vi "API Tree.vi"   [LabVIEW 2017]
uses:
  user.lib/_NEVSTOP/Communicable State Machine(CSM)/Communicable State Machine.lvlib
  examples/NEVSTOP/Communicable State Machine(CSM)/1. Create a reuse Module/1. Create a reuse Module.lvlib
  examples/NEVSTOP/Communicable State Machine(CSM)/4. Advance Examples/1. Action Workers Example/Action Worker Mode Example.lvlib
  examples/NEVSTOP/Communicable State Machine(CSM)/4. Advance Examples/3. Build-in Error Handling Framework/Build-in Error Handling Framework.lvlib
  examples/NEVSTOP/Communicable State Machine(CSM)/4. Advance Examples/2. Chain of Responsiblility Example/Chain of Responsibility Example.lvlib
  examples/NEVSTOP/Communicable State Machine(CSM)/4. Advance Examples/5. Multi-Loop Module Example/Multi-Loop Module Example.lvlib
  examples/NEVSTOP/Communicable State Machine(CSM)/4. Advance Examples/4. Global Log Filter Example/CSM Global Log Filter Example.lvlib
  user.lib/_NEVSTOP/Communicable State Machine(CSM)/_csmHelper/CSM-Helper.lvclass
  user.lib/_NEVSTOP/Communicable State Machine(CSM)/_csmHelper/lvcsmFile/lvcsm File Support.lvlib
  ddc9829f-1ac7-4767-a110-42ef600eb457.vi
  d8c6dec9-3888-43a3-80fe-73705555c2a7.vi
  user.lib/_NEVSTOP/Communicable State Machine(CSM)/_csmHelper/API with lvcsm Support/CSM-Helper API with lvcsm Support.lvlib
  user.lib/_NEVSTOP/Communicable State Machine(CSM)/_csmHelper/Utility/CSM-Helper Utility.lvlib
  user.lib/_NEVSTOP/Communicable State Machine(CSM)/_xnode/csm_tool/_xnode_csm_tool_support/CSM DebugTool Dialog.lvlib
  user.lib/_NEVSTOP/Communicable State Machine(CSM)/_quickdrop/CSM-QuickDrops.lvlib
  f0afa659-d9d9-457f-96a9-986d16a4897c.vi
  23e5c420-4285-4359-b20e-bc9ce14852c1.vi
  user.lib/_NEVSTOP/Communicable State Machine(CSM)/_Shared/CSM Shared.lvlib
  user.lib/_NEVSTOP/Communicable State Machine(CSM)/_csmHelper/Utility/Is CSM Module - VIRef.vi
  user.lib/_NEVSTOP/Communicable State Machine(CSM)/_Support/GlobalEvent/GEvt-Filter Global Log - v1.1.vi
  user.lib/_NEVSTOP/Communicable State Machine(CSM)/_Polymophic/CSM - Filter Local States.vi
  user.lib/_NEVSTOP/Communicable State Machine(CSM)/_Support/GlobalEvent/GEvt-Set Source Filter Rules - v1.0.vi
  user.lib/_NEVSTOP/Communicable State Machine(CSM)/_Support/GlobalEvent/GEvt-Convert Filter Rules - Periodic Setting Only.vi
  user.lib/_NEVSTOP/Communicable State Machine(CSM)/_csmHelper/API/Doc.vi
  user.lib/_NEVSTOP/Communicable State Machine(CSM)/_Polymophic/CSM - Filter Duplicated Lines.vi
  user.lib/_NEVSTOP/Communicable State Machine(CSM)/_Polymophic/Build Register Message.vi
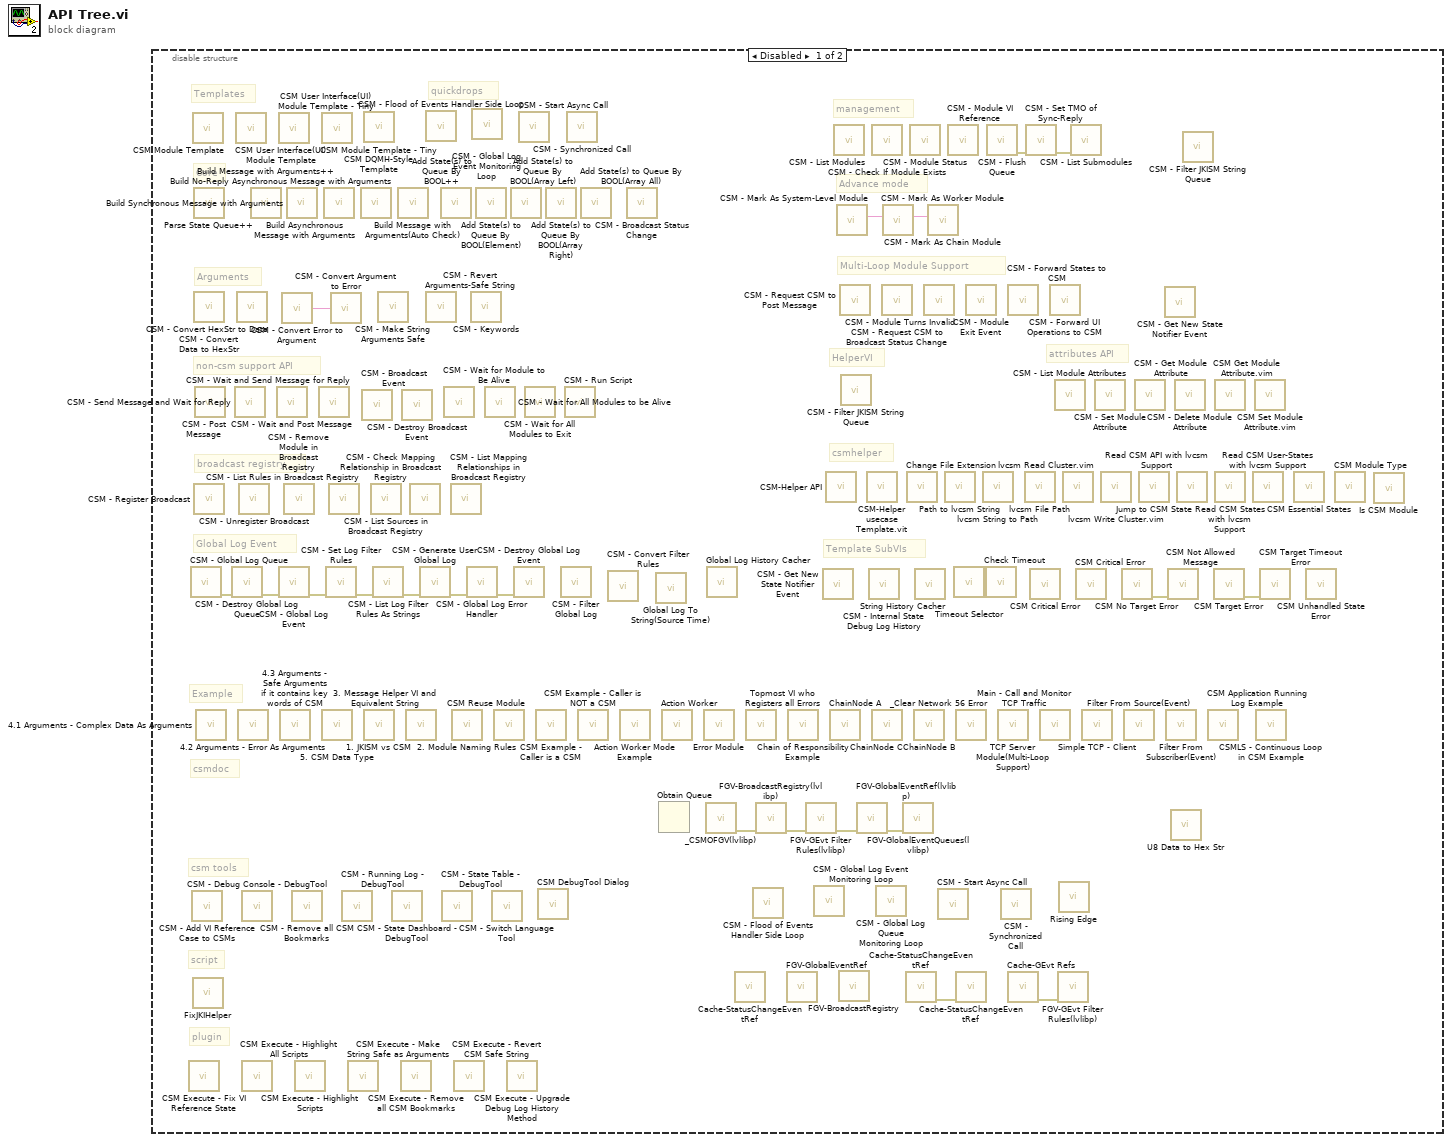
[diagram p0: block diagram]
diagram:
  n1 = disable-structure shown="Disabled" {
    frame Disabled {
      # "attributes API"
      # "management"
      # "Template SubVIs"
      # "Advance mode"
      # "broadcast registry"
      # "Core"
      # "Arguments"
      # "Global Log Event"
      # "HelperVI"
      # "Multi-Loop Module Support"
      # "Templates"
      # "non-csm support API"
      # "plugin"
      # "script"
      # "quickdrops"
      # "csm tools"
      # "csmhelper"
      # "csmdoc"
      # "Example"
      n2 = call "CSM Execute - Fix VI Reference State.vi"() -> ()  [unwired: 11 in, 1 out]
      n3 = call "CSM - Global Log Queue.vi"() -> ("error out"=w8:errorcluster)  [unwired: 10 in, 1 out]
      n4 = call "CSM - Add VI Reference Case to CSMs.vi"() -> ()  [unwired: 12 in]
      n5 = call "CSM Module Template.vi"() -> ()  [unwired: 12 in]
      n6 = call "FixJKIHelper.vi"() -> ()  [unwired: 12 in]
      n7 = call "Parse State Queue++.vi"() -> ()  [unwired: 10 in, 6 out]
      n8 = call "CSM - Convert Data to HexStr.vi"() -> ()  [unwired: 9 in, 1 out]
      n9 = call "CSM - Register Broadcast.vi"() -> ()  [unwired: 14 in, 2 out]
      n10 = call "CSM - Post Message.vi"() -> ()  [unwired: 11 in, 1 out]
      n11 = call "4.1 Arguments - Complex Data As Arguments.vi"() -> ()  [unwired: 12 in]
      n12 = call "CSM - Destroy Global Log Queue.vi"("Error In"=w8) -> ("error out"=w9:errorcluster)  [unwired: 10 in]
      n13 = call "CSM - Send Message and Wait for Reply.vi"() -> ()  [unwired: 9 in, 3 out]
      n14 = call "CSM User Interface(UI) Module Template.vi"() -> ()  [unwired: 12 in]
      n15 = call "CSM - Convert HexStr to Data.vi"() -> ()  [unwired: 8 in, 2 out]
      n16 = call "4.2 Arguments - Error As Arguments.vi"() -> ()  [unwired: 12 in]
      n17 = call "CSM - Unregister Broadcast.vi"() -> ()  [unwired: 14 in, 2 out]
      n18 = call "CSM - Debug Console - DebugTool.vi"() -> ()  [unwired: 12 in]
      n19 = call "CSM Execute - Highlight All Scripts.vi"() -> ()  [unwired: 11 in, 1 out]
      n20 = call-poly "Build Message with Arguments++.vi"() -> ()  [unwired: 15 in, 1 out]
      n21 = call "CSM - Wait and Post Message.vi"() -> ()  [unwired: 14 in, 2 out]
      n22 = call "CSM User Interface(UI) Module Template - Tiny.vi"() -> ()  [unwired: 12 in]
      n23 = call "CSM - Global Log Event.vi"("Error In"=w9) -> ("error out"=w20:errorcluster)  [unwired: 9 in, 1 out]
      n24 = call "4.3 Arguments - Safe Arguments if it contains key words of CSM.vi"() -> ()  [unwired: 12 in]
      n25 = call "CSM - Convert Error to Argument.vi"() -> ("Argument"=w15:string)  [unwired: 5 in]
      n26 = call "CSM - Remove Module in Broadcast Registry.vi"() -> ()  [unwired: 14 in, 2 out]
      n27 = call "Build Synchronous Message with Arguments.vi"() -> ()  [unwired: 15 in, 1 out]
      n28 = call "CSM - Remove all CSM Bookmarks.vi"() -> ()  [unwired: 12 in]
      n29 = call "CSM Execute - Highlight Scripts.vi"() -> ()  [unwired: 11 in, 1 out]
      n30 = call "CSM - Wait and Send Message for Reply.vi"() -> ()  [unwired: 12 in, 4 out]
      n31 = call "CSM Module Template - Tiny.vi"() -> ()  [unwired: 12 in]
      n32 = call "5. CSM Data Type.vi"() -> ()  [unwired: 12 in]
      n33 = call "Build Asynchronous Message with Arguments.vi"() -> ()  [unwired: 15 in, 1 out]
      n34 = call-poly "CSM - Set Log Filter Rules.vi"("Error In"=w20) -> ("error out"=w19:errorcluster)  [unwired: 10 in]
      n35 = call "CSM - List Rules in Broadcast Registry.vi"() -> ()  [unwired: 9 in, 3 out]
      n36 = call "CSM - Convert Argument to Error.vi"("Argument"=w15) -> ()  [unwired: 4 in, 1 out]
      n37 = call "CSM - Running Log - DebugTool.vi"() -> ()  [unwired: 12 in]
      n38 = call "CSM Execute - Make String Safe as Arguments.vi"() -> ()  [unwired: 11 in, 1 out]
      n39 = call "Build No-Reply Asynchronous Message with Arguments.vi"() -> ()  [unwired: 15 in, 1 out]
      n40 = call "CSM - Broadcast Event.vi"() -> ()  [unwired: 9 in, 3 out]
      n41 = call "CSM DQMH-Style Template.vi"() -> ()  [unwired: 12 in]
      n42 = call "1. JKISM vs CSM.vi"() -> ()  [unwired: 12 in]
      n43 = call "CSM - List Sources in Broadcast Registry.vi"() -> ()  [unwired: 10 in, 2 out]
      n44 = call "CSM - List Log Filter Rules As Strings.vi"("Error In"=w19) -> ("error out"=w18:errorcluster)  [unwired: 9 in, 1 out]
      n45 = call "CSM - Make String Arguments Safe.vi"() -> ()  [unwired: 9 in, 1 out]
      n46 = call "CSM - State Dashboard - DebugTool.vi"() -> ()  [unwired: 12 in]
      n47 = call "Build Message with Arguments(Auto Check).vi"() -> ()  [unwired: 15 in, 1 out]
      n48 = call "CSM Execute - Remove all CSM Bookmarks.vi"() -> ()  [unwired: 11 in, 1 out]
      n49 = call "CSM - Destroy Broadcast Event.vi"() -> ()  [unwired: 11 in, 1 out]
      n50 = call "3. Message Helper VI and Equivalent String.vi"() -> ()  [unwired: 12 in]
      n51 = call "CSM - Check Mapping Relationship in Broadcast Registry.vi"() -> ()  [unwired: 10 in, 2 out]
      n52 = call "CSM - Generate User Global Log.vi"("Error In"=w18) -> ("error out"=w17:errorcluster)  [unwired: 10 in]
      n53 = call "CSM - Flood of Events Handler Side Loop.vi"() -> ()  [unwired: 12 in]
      n54 = call "CSM - Revert Arguments-Safe String.vi"() -> ()  [unwired: 9 in, 1 out]
      n55 = call-poly "Add State(s) to Queue By BOOL++.vi"() -> ()  [unwired: 11 in, 1 out]
      n56 = call "CSM - State Table - DebugTool.vi"() -> ()  [unwired: 12 in]
      n57 = call "CSM - Wait for Module to Be Alive.vi"() -> ()  [unwired: 13 in, 3 out]
      n58 = call "CSM - List Mapping Relationships in Broadcast Registry.vi"() -> ()  [unwired: 10 in, 2 out]
      n59 = call "2. Module Naming Rules.vi"() -> ()  [unwired: 12 in]
      n60 = call "CSM Execute - Revert CSM Safe String.vi"() -> ()  [unwired: 11 in, 1 out]
      n61 = call "CSM - Global Log Error Handler.vi"("Error In"=w17) -> ("error out"=w16:errorcluster)  [unwired: 10 in]
      n62 = call "CSM - Keywords.vi"() -> ()  [unwired: 10 in, 2 out]
      n63 = call "CSM - Global Log Event Monitoring Loop.vi"() -> ()  [unwired: 12 in]
      n64 = call "Add State(s) to Queue By BOOL(Element).vi"() -> ()  [unwired: 11 in, 1 out]
      n65 = call "CSM - Wait for All Modules to be Alive.vi"() -> ()  [unwired: 9 in, 3 out]
      n66 = call "CSM - Switch Language Tool.vi"() -> ()  [unwired: 12 in]
      n67 = call "CSM Reuse Module.vi"() -> ()  [unwired: 12 in]
      n68 = call "CSM Execute - Upgrade Debug Log History Method.vi"() -> ()  [unwired: 11 in, 1 out]
      n69 = call "Add State(s) to Queue By BOOL(Array Left).vi"() -> ()  [unwired: 11 in, 1 out]
      n70 = call "CSM - Destroy Global Log Event.vi"("Error In"=w16) -> ()  [unwired: 10 in, 1 out]
      n71 = call "CSM - Start Async Call.vi"() -> ()  [unwired: 12 in]
      n72 = call "CSM - Wait for All Modules to Exit.vi"() -> ()  [unwired: 9 in, 3 out]
      n73 = call "CSM Example - Caller is a CSM.vi"() -> ()  [unwired: 12 in]
      n74 = call "CSM DebugTool Dialog.vi"() -> ()  [unwired: 12 in]
      n75 = call "Add State(s) to Queue By BOOL(Array Right).vi"() -> ()  [unwired: 11 in, 1 out]
      n76 = call-poly "CSM - Filter Global Log.vi"() -> ()  [unwired: 9 in, 3 out]
      n77 = call "CSM - Run Script.vi"() -> ()  [unwired: 13 in, 3 out]
      n78 = call "CSM - Synchronized Call.vi"() -> ()  [unwired: 12 in]
      n79 = call "CSM Example - Caller is NOT a CSM.vi"() -> ()  [unwired: 12 in]
      n80 = call "Add State(s) to Queue By BOOL(Array All).vi"() -> ()  [unwired: 11 in, 1 out]
      n81 = call-poly "CSM - Convert Filter Rules.vi"() -> ()  [unwired: 11 in, 1 out]
      n82 = call "Action Worker Mode Example.vi"() -> ()  [unwired: 12 in]
      n83 = call "CSM - Broadcast Status Change.vi"() -> ()  [unwired: 15 in, 1 out]
      n84 = call "Global Log To String(Source Time).vi"() -> ()  [unwired: 10 in, 1 out]
      n85 = Obtain Queue() -> ()  [unwired: 5 in, 3 out]
      n86 = call "Action Worker.vi"() -> ()  [unwired: 12 in]
      n87 = call "Error Module.vi"() -> ()  [unwired: 12 in]
      n88 = call "_CSMOFGV(lvlibp).vi"() -> ("error out"=w5:errorcluster)  [unwired: 9 in, 2 out]
      n89 = call "Global Log History Cacher.vi"() -> ()  [unwired: 15 in, 1 out]
      n90 = call "Cache-StatusChangeEventRef.vi"() -> ()  [unwired: 9 in, 3 out]
      n91 = call "Topmost VI who Registers all Errors.vi"() -> ()  [unwired: 12 in]
      n92 = call "CSM - Flood of Events Handler Side Loop.vi"() -> ()  [unwired: 12 in]
      n93 = call "FGV-BroadcastRegistry(lvlibp).vi"("Error In"=w5) -> ("error out"=w4:errorcluster)  [unwired: 12 in, 2 out]
      n94 = call "FGV-GlobalEventRef.vi"() -> ()  [unwired: 10 in, 2 out]
      n95 = call "Chain of Responsibility Example.vi"() -> ()  [unwired: 12 in]
      n96 = call "FGV-GEvt Filter Rules(lvlibp).vi"("Error In"=w4) -> ("error out"=w3:errorcluster)  [unwired: 9 in, 1 out]
      n97 = call "CSM - Global Log Event Monitoring Loop.vi"() -> ()  [unwired: 12 in]
      n98 = call "CSM - Get New State Notifier Event.vi"() -> ()  [unwired: 10 in, 2 out]
      n99 = call-poly "CSM-Helper API.vi"() -> ()  [unwired: 8 in, 4 out]
      n100 = call "ChainNode A.vi"() -> ()  [unwired: 12 in]
      n101 = call "CSM - List Modules.vi"() -> ()  [unwired: 10 in, 2 out]
      n102 = call "CSM - Mark As System-Level Module.vi"() -> ("CSM Name (Marked As Sysetem-Level Module)"=w14:string)  [unwired: 10 in]
      n103 = call "FGV-BroadcastRegistry.vi"() -> ()  [unwired: 13 in, 3 out]
      n104 = call "CSM - Request CSM to Post Message.vi"() -> ()  [unwired: 11 in, 1 out]
      n105 = call-poly "CSM - Filter JKISM String Queue.vi"() -> ()  [unwired: 15 in, 1 out]
      n106 = call "FGV-GlobalEventRef(lvlibp).vi"("error in (no error)"=w3) -> ("error out"=w2:errorcluster)  [unwired: 9 in, 1 out]
      n107 = call "CSM-Helper usecase Template.vit"() -> ()  [unwired: 10 in, 2 out]
      n108 = call "CSM - Internal State Debug Log History.vi"() -> ()  [unwired: 15 in, 1 out]
      n109 = call "CSM - Check If Module Exists.vi"() -> ()  [unwired: 9 in, 3 out]
      n110 = call "ChainNode C.vi"() -> ()  [unwired: 12 in]
      n111 = call "CSM - Global Log Queue Monitoring Loop.vi"() -> ()  [unwired: 12 in]
      n112 = call "CSM - Request CSM to Broadcast Status Change.vi"() -> ()  [unwired: 11 in, 1 out]
      n113 = call "CSM - Mark As Worker Module.vi"("CSM Name"=w14) -> ("CSM Name (Marked As Worker)"=w13:string)  [unwired: 9 in]
      n114 = call "FGV-GlobalEventQueues(lvlibp).vi"("error in (no error)"=w2) -> ()  [unwired: 8 in, 3 out]
      n115 = call "Cache-StatusChangeEventRef.vi"() -> ("error out"=w7:errorcluster)  [unwired: 9 in, 2 out]
      n116 = call "Change File Extension.vi"() -> ()  [unwired: 10 in, 2 out]
      n117 = call "CSM - Module Status.vi"() -> ()  [unwired: 7 in, 5 out]
      n118 = call "ChainNode B.vi"() -> ()  [unwired: 12 in]
      n119 = call "String History Cacher.vi"() -> ()  [unwired: 11 in, 1 out]
      n120 = call "CSM - Module Turns Invalid.vi"() -> ()  [unwired: 3 in, 1 out]
      n121 = call "CSM - Mark As Chain Module.vi"("CSM Name"=w13) -> ()  [unwired: 9 in, 1 out]
      n122 = call "CSM - Start Async Call.vi"() -> ()  [unwired: 12 in]
      n123 = call "Path to lvcsm String.vi"() -> ()  [unwired: 11 in, 1 out]
      n124 = call "CSM - Module VI Reference.vi"() -> ()  [unwired: 10 in, 2 out]
      n125 = call "Timeout Selector.vi"() -> ()  [unwired: 7 in, 1 out]
      n126 = call "_Clear Network 56 Error.vi"() -> ()  [unwired: 5 in, 1 out]
      n127 = call "Cache-StatusChangeEventRef.vi"("error in (no error)"=w7) -> ()  [unwired: 8 in, 3 out]
      n128 = call "CSM - Module Exit Event.vi"() -> ()  [unwired: 9 in, 3 out]
      n129 = call "lvcsm String to Path.vi"() -> ()  [unwired: 11 in, 1 out]
      n130 = call "Check Timeout.vi"() -> ()  [unwired: 8 in, 1 out]
      n131 = call "CSM - Flush Queue.vi"() -> ("error out"=w10:errorcluster)  [unwired: 9 in, 2 out]
      n132 = call "TCP Server Module(Multi-Loop Support).vi"() -> ()  [unwired: 12 in]
      n133 = call "CSM - Synchronized Call.vi"() -> ()  [unwired: 12 in]
      n134 = call "CSM - Forward States to CSM.vi"() -> ()  [unwired: 11 in, 1 out]
      n135 = call "Cache-GEvt Refs.vi"() -> ("error out"=w6:errorcluster)  [unwired: 10 in, 1 out]
      n136 = call "lvcsm File Path.vi"() -> ()  [unwired: 3 in, 1 out]
      n137 = call "CSM - Set TMO of Sync-Reply.vi"("Error In"=w10) -> ("error out"=w1:errorcluster)  [unwired: 9 in, 1 out]
      n138 = call "CSM Critical Error.vi"() -> ()  [unwired: 11 in, 1 out]
      n139 = call "Main - Call and Monitor TCP Traffic.vi"() -> ()  [unwired: 12 in]
      n140 = call "CSM - Forward UI Operations to CSM.vi"() -> ()  [unwired: 10 in, 2 out]
      n141 = call "CSM - List Module Attributes.vi"() -> ()  [unwired: 11 in, 5 out]
      n142 = call "FGV-GEvt Filter Rules(lvlibp).vi"("Error In"=w6) -> ()  [unwired: 9 in, 2 out]
      n143 = call "Rising Edge.vi"() -> ()  [unwired: 1 in, 1 out]
      n144 = call "lvcsm Read Cluster.vim"() -> ()  [unwired: 10 in, 2 out]
      n145 = call "CSM - List Submodules.vi"("Error In"=w1) -> ()  [unwired: 8 in, 3 out]
      n146 = call "CSM Critical Error.vi"() -> ()  [unwired: 11 in, 1 out]
      n147 = call "Simple TCP - Client.vi"() -> ()  [unwired: 12 in]
      n148 = call "CSM - Set Module Attribute.vi"() -> ()  [unwired: 12 in, 4 out]
      n149 = call "lvcsm Write Cluster.vim"() -> ()  [unwired: 11 in, 1 out]
      n150 = call "CSM No Target Error.vi"() -> ("error out"=w12:errorcluster)  [unwired: 11 in]
      n151 = call "Filter From Source(Event).vi"() -> ()  [unwired: 12 in]
      n152 = call "CSM - Get Module Attribute.vi"() -> ()  [unwired: 11 in, 5 out]
      n153 = call "Jump to CSM State.vi"() -> ()  [unwired: 11 in, 1 out]
      n154 = call "CSM - Get New State Notifier Event.vi"() -> ()  [unwired: 10 in, 2 out]
      n155 = call "Filter From Subscriber(Event).vi"() -> ()  [unwired: 12 in]
      n156 = call "CSM Not Allowed Message.vi"("error in (no error)"=w12) -> ()  [unwired: 10 in, 1 out]
      n157 = call "U8 Data to Hex Str.vi"() -> ()  [unwired: 1 in, 1 out]
      n158 = call "CSM - Delete Module Attribute.vi"() -> ()  [unwired: 12 in, 4 out]
      n159 = call "Read CSM API with lvcsm Support.vi"() -> ()  [unwired: 10 in, 2 out]
      n160 = call-poly "CSM - Filter JKISM String Queue.vi"() -> ()  [unwired: 15 in, 1 out]
      n161 = call "CSM Application Running Log Example.vi"() -> ()  [unwired: 12 in]
      n162 = call "CSM Target Error.vi"() -> ("error out"=w11:errorcluster)  [unwired: 11 in]
      n163 = call "CSM Get Module Attribute.vim"() -> ()  [unwired: 11 in, 5 out]
      n164 = call "Read CSM States with lvcsm Support.vi"() -> ()  [unwired: 10 in, 2 out]
      n165 = call "Read CSM User-States with lvcsm Support.vi"() -> ()  [unwired: 10 in, 2 out]
      n166 = call "CSM Set Module Attribute.vim"() -> ()  [unwired: 12 in, 4 out]
      n167 = call "CSMLS - Continuous Loop in CSM Example.vi"() -> ()  [unwired: 12 in]
      n168 = call "CSM Target Timeout Error.vi"("error in (no error)"=w11) -> ()  [unwired: 10 in, 1 out]
      n169 = call "CSM Essential States.vi"() -> ()  [unwired: 11 in, 1 out]
      n170 = call "CSM Unhandled State Error.vi"() -> ()  [unwired: 11 in, 1 out]
      n171 = call "CSM Module Type.vi"() -> ()  [unwired: 9 in, 3 out]
      n172 = call-poly "Is CSM Module.vi"() -> ()  [unwired: 8 in, 4 out]
    }
    frame Enabled {
    }
  }
